vi "waveformgraph_wdt.vi"() -> ()   [LabVIEW 2023]
panel:
  in  "x1":dbl
  out "Waveform_Graph_As_WDT":waveform(dbl)(graph)
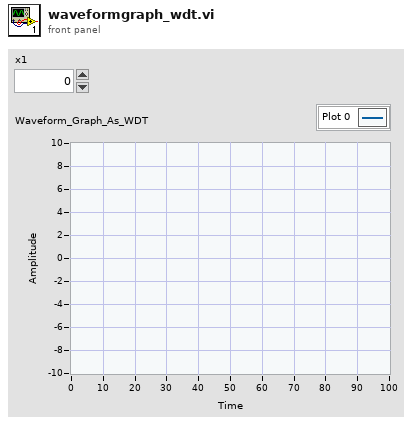
[diagram p1: front panel]
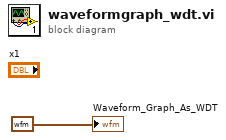
[diagram p0: block diagram]
diagram:
  "Waveform_Graph_As_WDT" <- waveform(dbl) {"t0"=timestamp(0 s since 1904-01-01), "dt"=1.0, "Y"=[]} ("Waveform")
